vi "GFITS_GetHdrType.vi"(10 "keyval":string) -> (1 "type":string, 2 "keyval out":string)   [LabVIEW 2016]
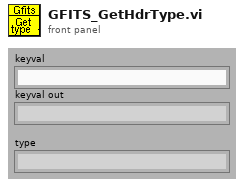
[diagram p1: front panel]
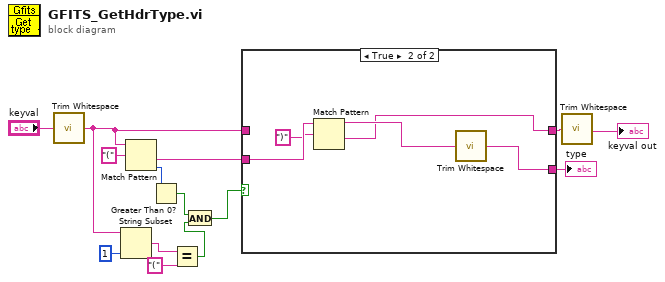
[diagram p0: block diagram]
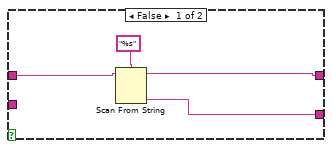
[diagram p2: hidden frame]
diagram:
  n1 = call <vilib>:"Trim Whitespace.vi"("string"="keyval") -> ("trimmed string"=w6:string)  [unwired: 1 in]
  n2 = String Subset(string=w6, length (rest)=1 ("length (rest)")) -> (substring=w3:string)  [unwired: 1 out]
  n3 = Match Pattern(string=w6, regular expression="(") -> (after substring=w13:string, offset past match=w12:i32)  [unwired: 3 out]
  n4 = Greater Than 0?(x=w12) -> (x > 0?=w8:bool)
  n5 = Equal?(x=w3, y="(") -> (x = y?=w4:bool)
  n6 = And(x=w8, y=w4) -> (x .and. y?=w1:bool)
  n7 = case shown="True" w1 {
    tunnel: w13 -> [_ w23]
    tunnel: w6 -> [w17 _]
    tunnel: [w15 w19] -> w11
    tunnel: [w16 w21] -> w10
    frame False {
      n8 = Scan From String(format string="%s" ("Format String"), input string=w17) -> (remaining string=w15:string, output 1=w16:string)  [unwired: 2 in, 3 out]
    }
    frame True {
      n9 = Match Pattern(string=w23, regular expression=")") -> (before substring=w20:string, after substring=w19:string)  [unwired: 3 out]
      n10 = call <vilib>:"Trim Whitespace.vi"("string"=w20) -> ("trimmed string"=w21:string)  [unwired: 1 in]
    }
  }
  "type" <- w10
  n11 = call <vilib>:"Trim Whitespace.vi"("string"=w11) -> ("trimmed string"=→"keyval out":string)  [unwired: 1 in]
